vi "Auto Balance Control DAO.vi"(7 "refnum":T1, 8 "error in (no error)":errorcluster, 10 "Autobalance Control In":T2={"Number of Samples"=0, "Delay After Cmd"=0, "Maximum Command"=0.0, "1/4 Linear Range"=0.5}, 11 "Persistent DAO Actions":T3) -> (0 "error out":errorcluster, 2 "Autobalance Control Out":T2={"Number of Samples"=0, "Delay After Cmd"=0, "Maximum Command"=0.0, "1/4 Linear Range"=0.5}, 4 "refnum out":T1)   [LabVIEW 2009]
uses:
  Metadata/Persistant DAO Actions.ctl
  Autobalance Control Parameters.ctl
  <vilib>/Utility/config.llb/Config Data RefNum.ctl
  <vilib>/Utility/config.llb/Read Key (Double).vi
  <vilib>/Utility/config.llb/Read Key (I32).vi
  <vilib>/Utility/config.llb/Read Key (U32).vi
  <vilib>/Utility/config.llb/Write Key (Double).vi
  <vilib>/Utility/config.llb/Write Key (I32).vi
  <vilib>/Utility/config.llb/NI_LVConfig.lvlib
panel:
  # "(Volts)"
  # "(Volts)"
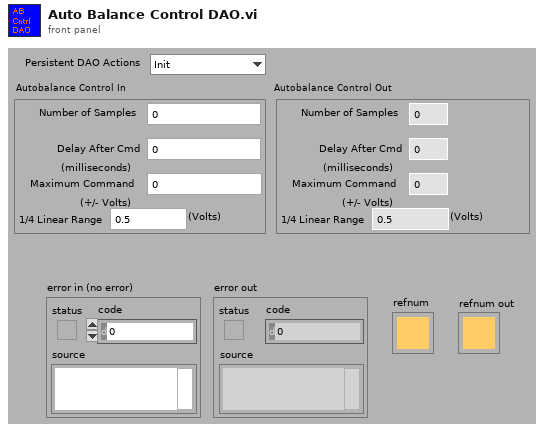
[diagram p1: front panel]
types:
  T1 = typedef "NI_LVConfig.lvlib/Config Data RefNum.ctl" = refnum<k1>
  T2 = typedef "Autobalance Control Parameters.ctl" = cluster{"Number of Samples":i32, "Delay After Cmd":i32, "Maximum Command":dbl, "1/4 Linear Range":dbl}
  T3 = typedef "Persistant DAO Actions.ctl" = enum16{"Init", "Get", "Set", "Load", "Save"}
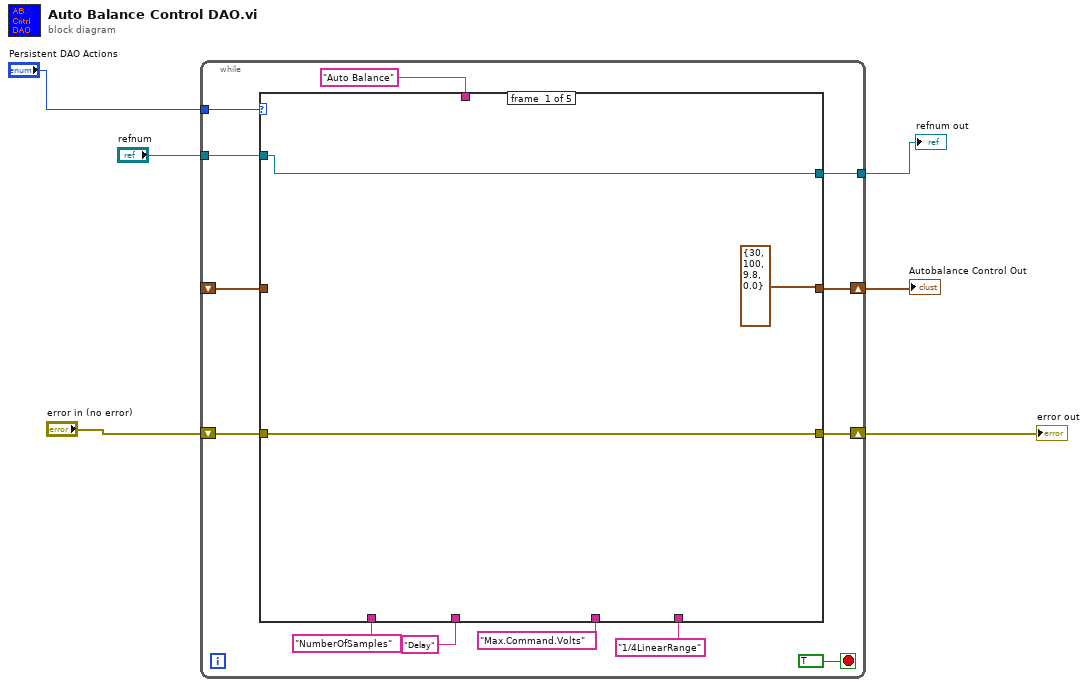
[diagram p0: block diagram]
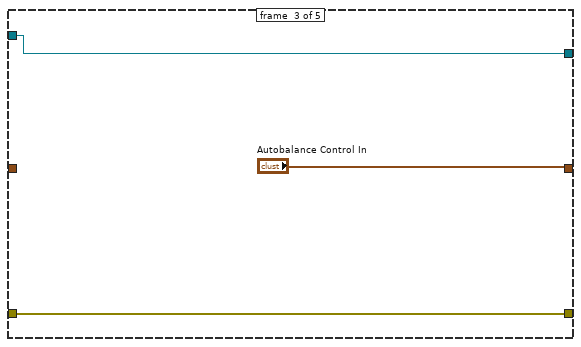
[diagram p3: hidden frame]
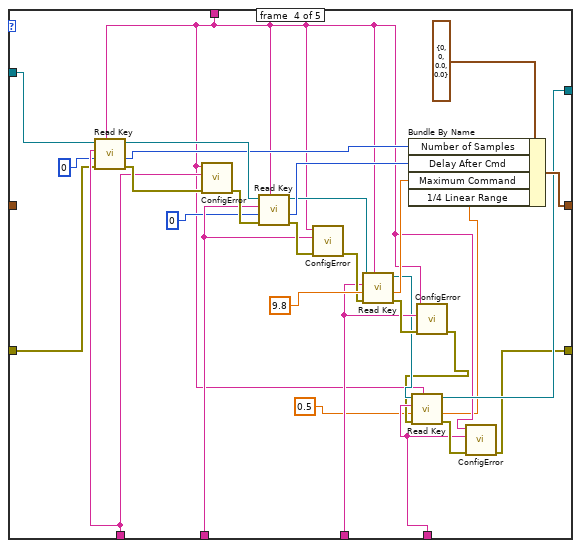
[diagram p4: hidden frame]
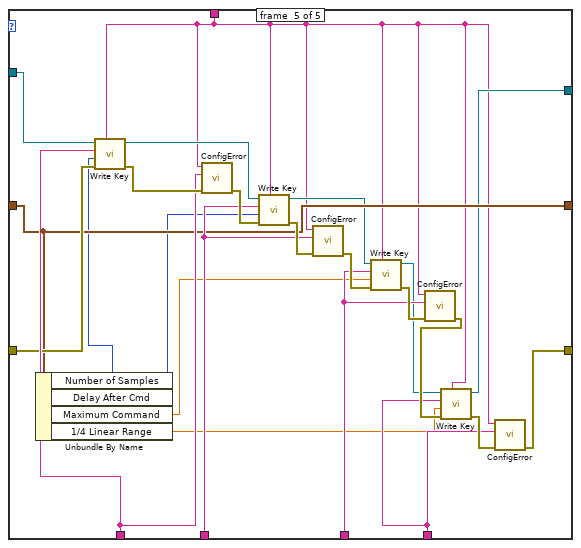
[diagram p5: hidden frame]
diagram:
  n1 = while {
    tunnel: "Persistent DAO Actions" -> [w18]
    shift-right: [w9] -> w5
    shift-left: _ -> [w10]
    tunnel: "refnum" -> [w15]
    shift-right: [w12] -> w2
    shift-left: "error in (no error)" -> [w13]
    tunnel: [w11] -> w1
    stop <- TRUE stop-if-true
    n2 = case shown="\"Load\"" w18 {
      tunnel: "Auto Balance" -> [_ _ _ w30 w58]
      tunnel: "NumberOfSamples" -> [_ _ _ w56 w80]
      tunnel: w15 -> [w22 w24 w27 w55 w79]
      tunnel: "Delay" -> [_ _ _ w51 w75]
      tunnel: w13 -> [w21 w25 w28 w49 w74]
      tunnel: [w21 w25 w28 w32 w63] -> w12
      tunnel: [w22 w24 w27 w34 w59] -> w11
      tunnel: w10 -> [_ w23 _ _ w73]
      tunnel: [T2 {"Number of Samples"=30, "Delay After Cmd"=100, "Maximum Command"=9.8, "1/4 Linear Range"=0.0} ("Autobalance Control In") w23 "Autobalance Control In" w44 w73] -> w9
      tunnel: "Max.Command.Volts" -> [_ _ _ w39 w67]
      tunnel: "1/4LinearRange" -> [_ _ _ w36 w62]
      frame #0 {
      }
      frame #1 {
      }
      frame #2 {
      }
      frame #3 {
        n3 = call-poly <vilib>:"Read Key.vi"("section"=w30, "error in (no error)"=w49, "default value"=u16 0 ("Port Number In"), "key"=w56, "refnum"=w55) -> ("error out"=w57:errorcluster, "value"=w46:u32, "refnum out"=w52:T1)  [unwired: 4 out]
        n4 = call "ConfigError.vi"("error in (no error)"=w57, "Key"=w56, "Section"=w30) -> ("error out"=w53:errorcluster)  [unwired: 8 out]
        n5 = call-poly <vilib>:"Read Key.vi"("section"=w30, "error in (no error)"=w53, "default value"=0 ("Wait For Notification Timeout In"), "key"=w51, "refnum"=w52) -> ("error out"=w54:errorcluster, "value"=w45:i32, "refnum out"=w42:T1)  [unwired: 4 out]
        n6 = call "ConfigError.vi"("error in (no error)"=w54, "Key"=w51, "Section"=w30) -> ("error out"=w40:errorcluster)  [unwired: 8 out]
        n7 = call-poly <vilib>:"Read Key.vi"("section"=w30, "error in (no error)"=w40, "default value"=9.8, "key"=w39, "refnum"=w42) -> ("error out"=w43:errorcluster, "value"=w38:dbl, "refnum out"=w35:T1)  [unwired: 4 out]
        n8 = call "ConfigError.vi"("error in (no error)"=w43, "Key"=w39, "Section"=w30) -> ("error out"=w33:errorcluster)  [unwired: 8 out]
        n9 = call-poly <vilib>:"Read Key.vi"("section"=w30, "error in (no error)"=w33, "default value"=0.5, "key"=w36, "refnum"=w35) -> ("error out"=w37:errorcluster, "value"=w29:dbl, "refnum out"=w34:T1)  [unwired: 4 out]
        n10 = Bundle By Name(cluster=T2 {"Number of Samples"=0, "Delay After Cmd"=0, "Maximum Command"=0.0, "1/4 Linear Range"=0.0} ("Autobalance Control In"), "Number of Samples"=w46, "Delay After Cmd"=w45, "Maximum Command"=w38, "1/4 Linear Range"=w29) -> (w44:T2)
        n11 = call "ConfigError.vi"("error in (no error)"=w37, "Key"=w36, "Section"=w30) -> ("error out"=w32:errorcluster)  [unwired: 8 out]
      }
      frame #4 {
        n12 = Unbundle By Name(w73) -> ("Number of Samples"=w72:i32, "Delay After Cmd"=w71:i32, "Maximum Command"=w66:dbl, "1/4 Linear Range"=w61:dbl)
        n13 = call-poly <vilib>:"Write Key.vi"("section"=w58, "error in (no error)"=w74, "value"=w72, "key"=w80, "refnum"=w79) -> ("error out"=w81:errorcluster, "refnum out"=w76:T1)  [unwired: 5 out]
        n14 = call "ConfigError.vi"("error in (no error)"=w81, "Key"=w80, "Section"=w58) -> ("error out"=w77:errorcluster)  [unwired: 8 out]
        n15 = call-poly <vilib>:"Write Key.vi"("section"=w58, "error in (no error)"=w77, "value"=w71, "key"=w75, "refnum"=w76) -> ("error out"=w78:errorcluster, "refnum out"=w68:T1)  [unwired: 5 out]
        n16 = call "ConfigError.vi"("error in (no error)"=w78, "Key"=w75, "Section"=w58) -> ("error out"=w69:errorcluster)  [unwired: 8 out]
        n17 = call-poly <vilib>:"Write Key.vi"("section"=w58, "error in (no error)"=w69, "value"=w66, "key"=w67, "refnum"=w68) -> ("error out"=w70:errorcluster, "refnum out"=w60:T1)  [unwired: 3 in, 2 out]
        n18 = call "ConfigError.vi"("error in (no error)"=w70, "Key"=w67, "Section"=w58) -> ("error out"=w64:errorcluster)  [unwired: 8 out]
        n19 = call-poly <vilib>:"Write Key.vi"("section"=w58, "error in (no error)"=w64, "value"=w61, "key"=w62, "refnum"=w60) -> ("error out"=w65:errorcluster, "refnum out"=w59:T1)  [unwired: 3 in, 2 out]
        n20 = call "ConfigError.vi"("error in (no error)"=w65, "Key"=w62, "Section"=w58) -> ("error out"=w63:errorcluster)  [unwired: 8 out]
      }
    }
  }
  "error out" <- w2
  "Autobalance Control Out" <- w5
  "refnum out" <- w1
